vi "PH_IEEE1394Camera.State Configure.vi"(0 "VI in":refnum<vi>, 5 "error in (no error)":errorcluster) -> (14 "VI out":refnum<vi>, 16 "Session Out":T1, 18 "Cam Error":errorcluster, 19 "error out":errorcluster)   [LabVIEW 2014, in "PH_IEEE1394Camera.lvlib"]
uses:
  PH_IEEE1394Camera.lvlib
  <vilib>/userdefined/High Color/IMAQdx.ctl
  PH_Cam_BaseClass/PH_Cam_BaseClass.lvlib
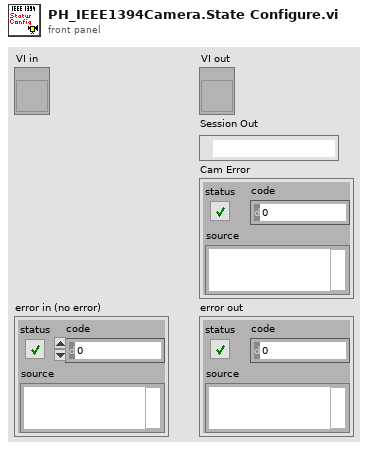
[diagram p1: front panel]
types:
  T1 = typedef "IMAQdx.ctl" = refnum<k21>
  T2 = typedef "PH_Cam_BaseClass.lvlib/PH_Cam_BaseClass.Settings.ctl" = cluster{"Cam ID":string, "Gain":dbl, "Brightness":dbl, "Shutter":dbl, "Mode":i32}
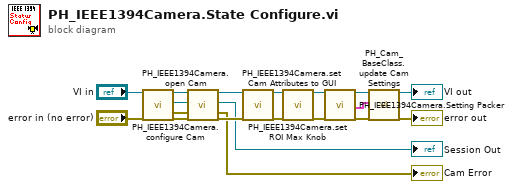
[diagram p0: block diagram]
diagram:
  n1 = call "PH_IEEE1394Camera.open Cam.vi"("VI in"="VI in", "error in (no error)"="error in (no error)") -> ("VI out"=w10:refnum<vi>, "Cam Session Out"=w8:T1, "Cam Error out"=w7:errorcluster, "error out"=w9:errorcluster)  [unwired: 14 in]
  n2 = call "PH_IEEE1394Camera.configure Cam.vi"("VI in"=w10, "IMAQ1394 Session In"=w8, "Cam Error in"=w7, "error in (no error)"=w9) -> ("VI out"=w4:refnum<vi>, "IMAQ1394 Session Out"=→"Session Out":T1, "Cam Error out"=→"Cam Error":errorcluster, "error out"=w3:errorcluster)  [unwired: 12 in]
  n3 = call "PH_IEEE1394Camera.set Cam Attributes to GUI.vi"("VI in"=w4, "error in (no error)"=w3) -> ("VI out"=w13:refnum<vi>, "error out"=w14:errorcluster)  [unwired: 16 in]
  n4 = call "PH_IEEE1394Camera.set ROI Max Knob.vi"("VI in"=w13, "error in (no error)"=w14) -> ("VI out"=w12:refnum<vi>, "error out"=w11:errorcluster)  [unwired: 16 in]
  n5 = call "PH_IEEE1394Camera.Setting Packer.vi"("i ref in"=w12, "error in (no error)"=w11) -> ("i ref out"=w16:refnum<vi>, "Cam Settings"=w15:T2, "error out"=w17:errorcluster)  [unwired: 15 in]
  n6 = call "PH_Cam_BaseClass.update Cam Settings.vi"("VI in"=w16, "Cam Settings In"=w15, "error in (no error)"=w17) -> ("VI out"=→"VI out":refnum<vi>, "error out"=→"error out":errorcluster)  [unwired: 15 in]
